vi "LinearPlntInvFF_Calculate.vi"(9 "NextR":T1, 10 "R":T1, 11 "Input Linear Plant Inv FF":T2) -> (0 "Error":bool, 2 "Uff":T1, 3 "Output Linear Plant Inv FF":T2)   [LabVIEW 2019, in "Trajectory_Library.lvlib"]
doc: "Creates a new LINEAR PLANT INVERSION FEEDFORWARD data cluster with the specified values. \n\n\nInputs: \n - XXX -- XXX.\n\nOutputs:\n - XXX -- XXX."
uses:
  Trajectory_Library.lvlib
  LINEAR_PLANT_INV_FF.ctl
  <vilib>/Analysis/Matrix/Datatypes/RealMatrix.ctl
  <vilib>/Analysis/baseanly.llb/Real A x B.vi
  <vilib>/Analysis/Matrix/Numeric/Subtract/Subtract - RM,RM.vi
  <vilib>/Analysis/7linalg.llb/Solve Linear Equations (multiple right hand).vi
  <vilib>/Analysis/Matrix/NI_Matrix.lvlib
  <vilib>/Analysis/NI_AALBase.lvlib
  <vilib>/Analysis/NI_AALPro.lvlib
panel:
  # "<States,1>"
  # "<Inputs,1>"
  # "<States,Inputs>"
  # "<States,States>"
  # "<States,1>"
  # "<Inputs,1>"
  # "<States,Inputs>"
  # "<States,States>"
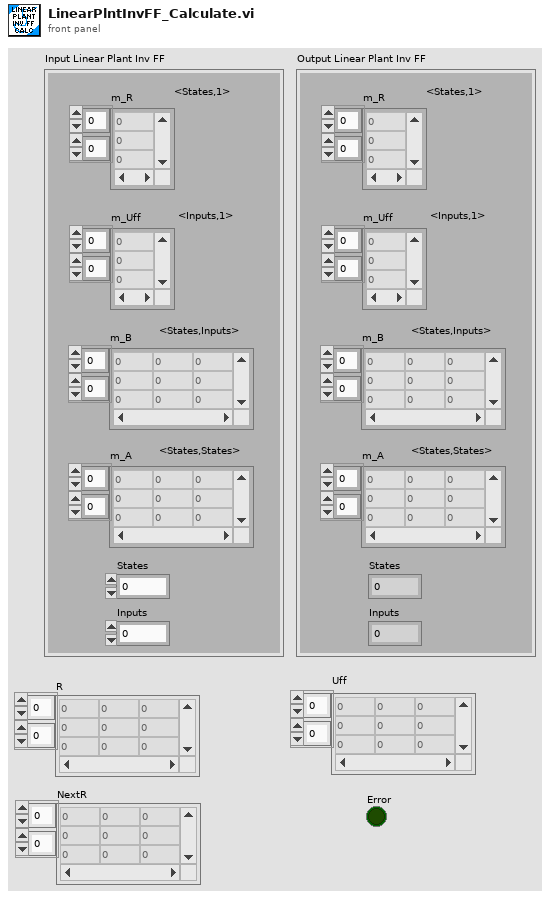
[diagram p1: front panel]
types:
  T1 = typedef "NI_Matrix.lvlib/RealMatrix.ctl" = dbl[][]
  T2 = typedef "Trajectory_Library.lvlib/LINEAR_PLANT_INV_FF.ctl" = cluster{"m_R":T1, "m_Uff":T1, "m_B":T1, "m_A":T1, "States":i32, "Inputs":i32}
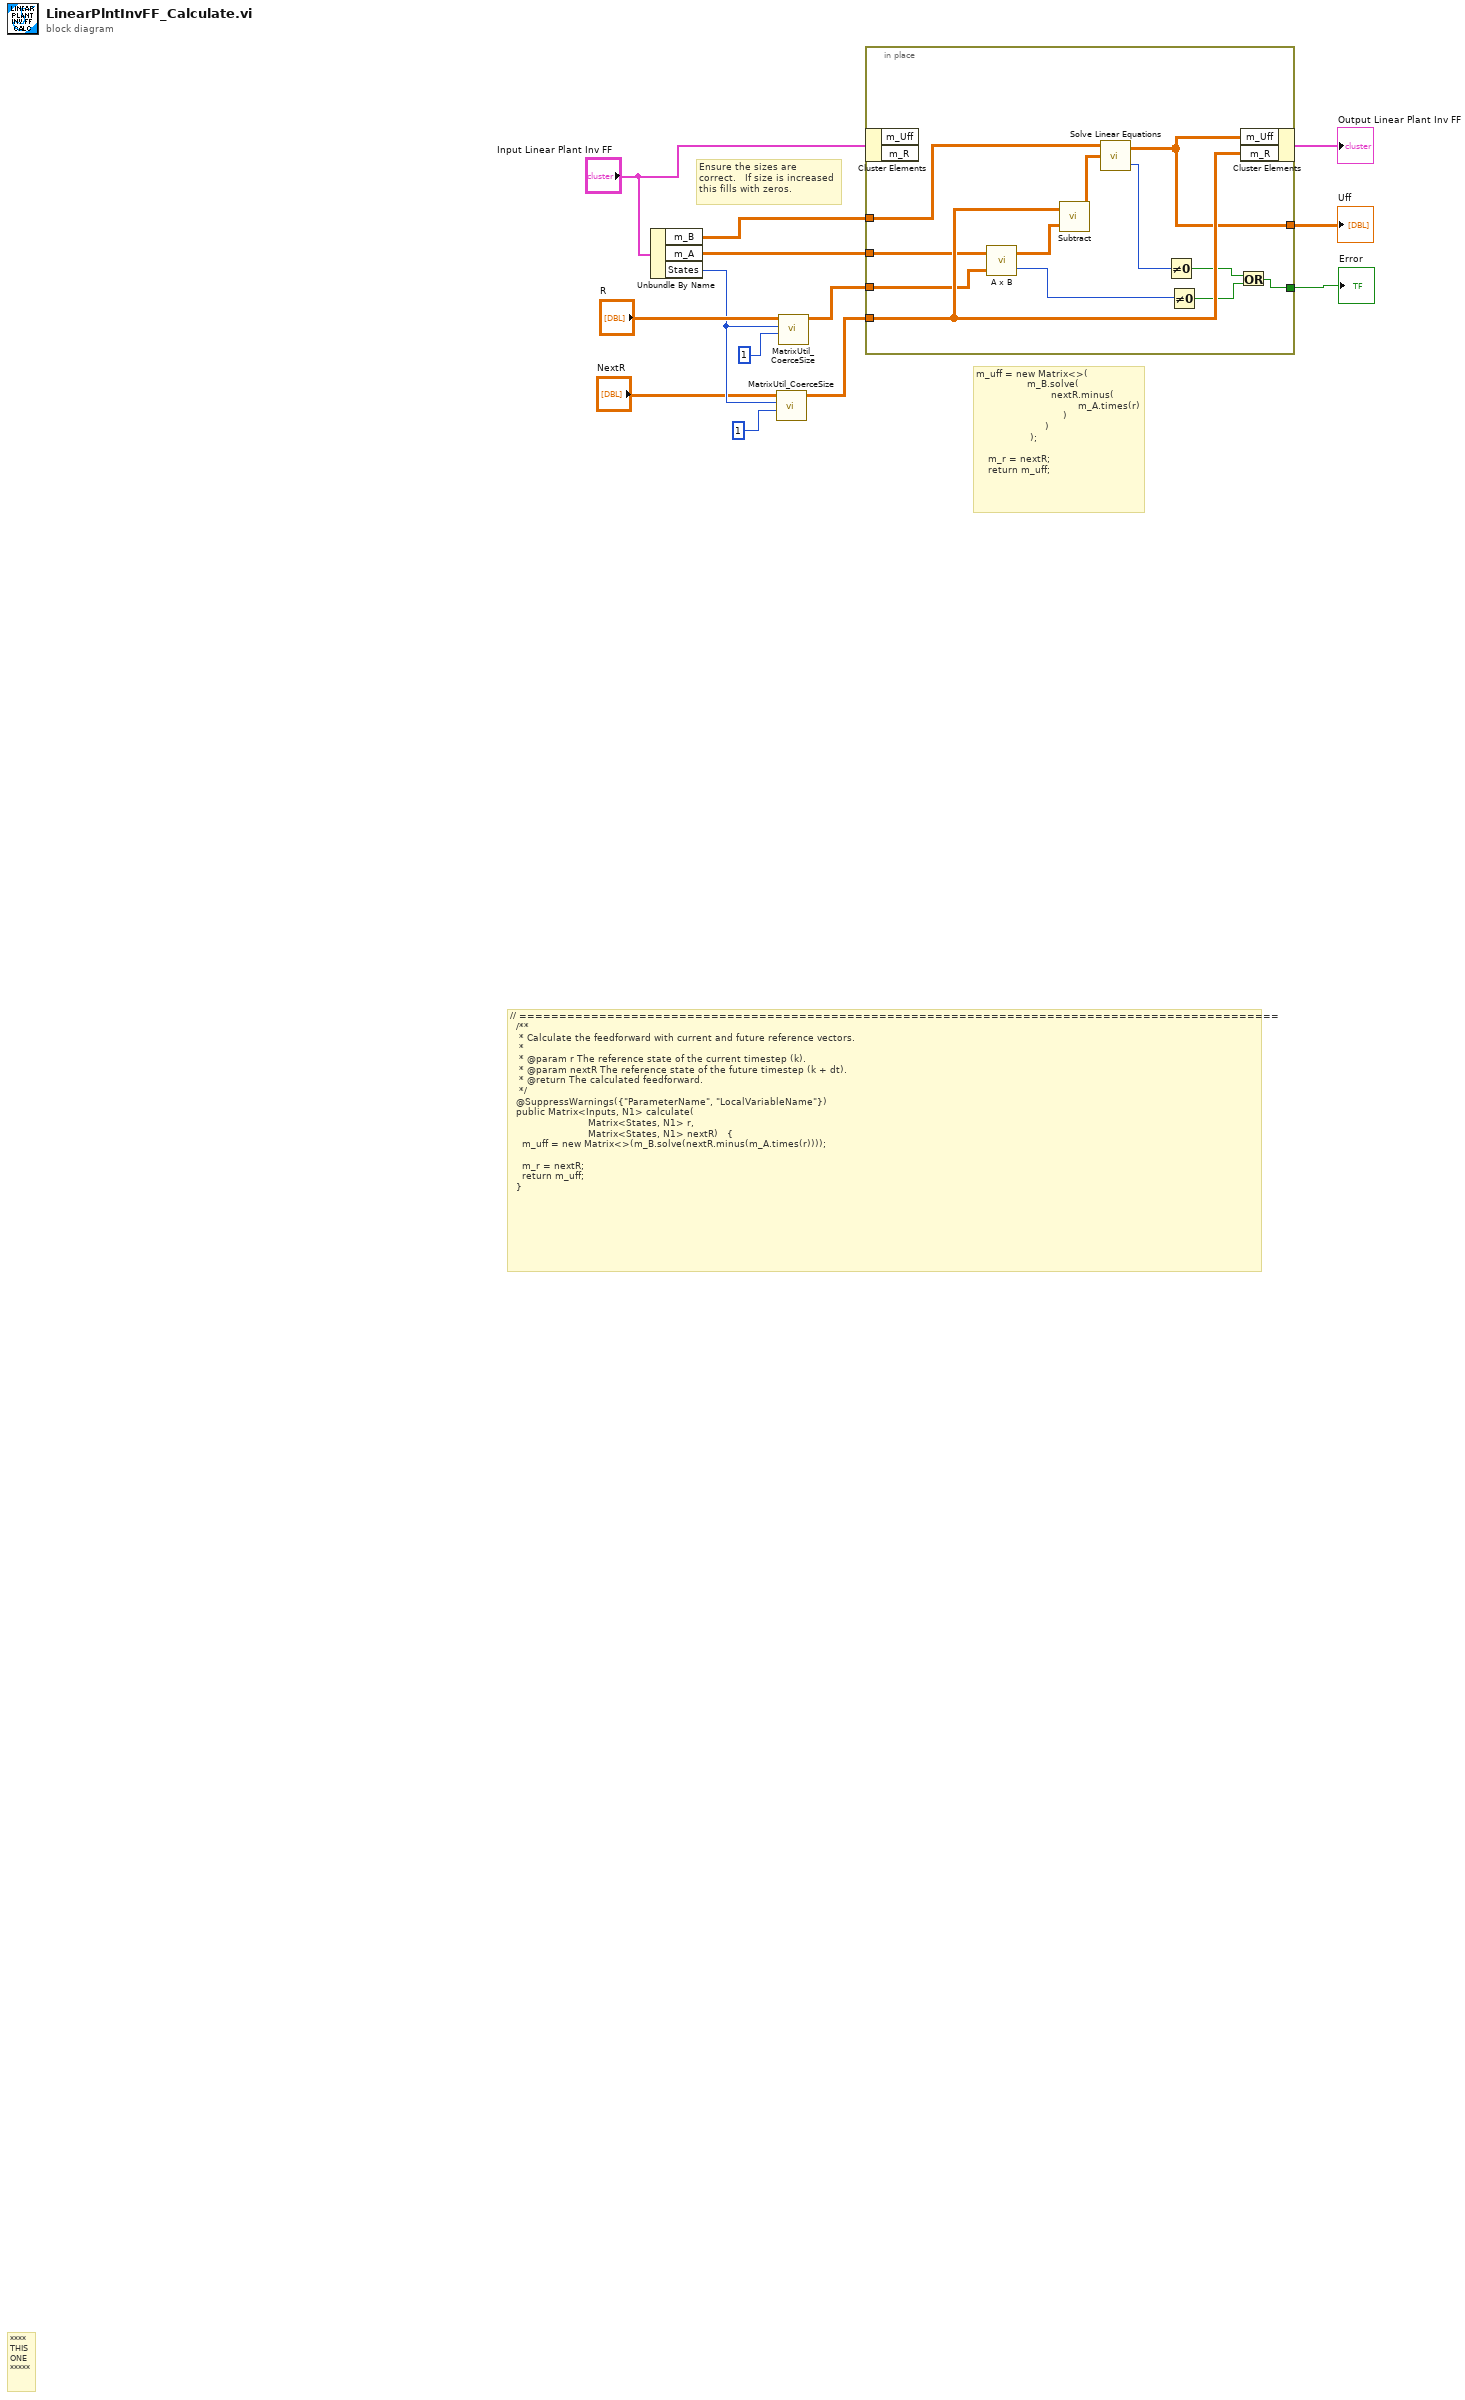
[diagram p0: block diagram]
diagram:
  # "m_uff = new Matrix<>(\n                 m_B.solve(\n                         nextR.minus(\n                                  m_A.times(r) \n                             )\n                       )\n                  );\n\n    m_r = nextR;\n    return m_uff;"
  # "// ===============================================================================================\n  /**\n   * Calculate the feedforward with current and future reference vectors.\n   *\n   * @param r The reference state of the current timestep (k).\n   * @param nextR The reference state of the future timestep (k + dt).\n   * @return The calculated feedforward.\n   */\n  @SuppressWarnings({\"ParameterName\", \"LocalVariableName\"})\n  public Matrix<Inputs, N1> calculate(\n                          Matrix<States, N1> r, \n                          Matrix<States, N1> nextR)   {\n    m_uff = new Matrix<>(m_B.solve(nextR.minus(m_A.times(r))));\n\n    m_r = nextR;\n    return m_uff;\n  }"
  # "Ensure the sizes are\ncorrect.   If size is increased \nthis fills with zeros."
  # "****\nTHIS\nONE\n*****"
  n1 = Unbundle By Name("Input Linear Plant Inv FF") -> ("m_B"=w11:T1, "m_A"=w12:T1, "States"=w4:i32)
  n2 = call "MatrixUtil_CoerceSize.vi"("Columns"=1 ("y"), "Rows"=w4, "input matrix"="NextR") -> ("output matrix"=w1:T1)  [unwired: 8 in]
  n3 = call "MatrixUtil_CoerceSize.vi"("Columns"=1 ("y"), "Rows"=w4, "input matrix"="R") -> ("output matrix"=w5:T1)  [unwired: 8 in]
  n4 = in-place {
    in-place-border: w1 -> [w25]
    in-place-border: w12 -> [w24]
    in-place-border: w5 -> [w23]
    in-place-border: w11 -> [w20]
    in-place-border: [w19] -> w9
    in-place-border: [w14] -> w8
    n5 = in-place-cluster #1("Input Linear Plant Inv FF") -> ()  [unwired: 2 out]
    n6 = call-poly <vilib>:"A x B.vi"("B"=w23, "A"=w24) -> ("error"=w18:i32, "A x B"=w22:T1)
    n7 = call-poly <vilib>:"Subtract.vi"("Real Matrix B"=w22, "Real Matrix A"=w25) -> ("A - B"=w21:T1)
    n8 = call-poly <vilib>:"Solve Linear Equations.vi"("Known Matrix"=w21, "Input Matrix"=w20) -> ("error"=w17:i32, "Solution Matrix"=w19:T1)  [unwired: 1 in]
    n9 = Not Equal To 0?(x=w17) -> (x != 0?=w16:bool)
    n10 = Not Equal To 0?(x=w18) -> (x != 0?=w15:bool)
    n11 = Or(x=w16, y=w15) -> (x .or. y?=w14:bool)
    n12 = in-place-cluster #1("m_Uff"=w19, "m_R"=w25) -> (→"Output Linear Plant Inv FF":T2)
  }
  "Uff" <- w9
  "Error" <- w8
